vi "Log DB.vi"(8 "error in (no error)":errorcluster, 11 "Class 2 in":refnum<class "Class 2.lvclass">) -> (0 "error out":errorcluster, 3 "Class 2 out":refnum<class "Class 2.lvclass">)   [LabVIEW 2019, in "Class 2.lvclass"]
uses:
  Class 2.lvclass
  Class 2.lvclass/Class 2.ctl
  <vilib>/addons/database/Connection.llb/DB Tools Open Connec (Path).vi
  <vilib>/addons/database/NI_Database_API.lvlib
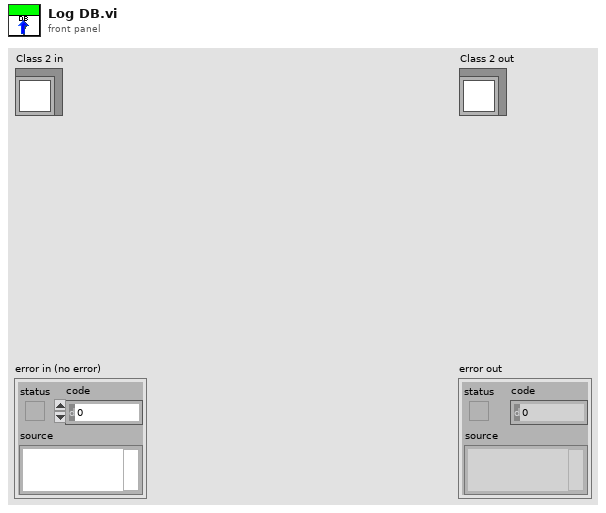
[diagram p1: front panel]
types:
  T1 = cluster{"Modelo":string, "date/time string":string, "Dato1":string, "Dato2":dbl}
  T2 = typedef "NI_Database_API.lvlib/Conn ObjectReference.ctl" = refnum<k1>
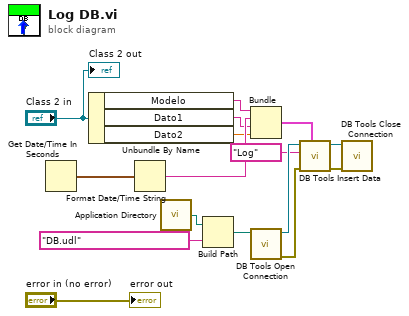
[diagram p0: block diagram]
diagram:
  n1 = Get Date/Time In Seconds() -> (seconds since 1Jan1904=w15:timestamp)
  n2 = Unbundle By Name("Class 2 in") -> ("Modelo"=w3:string, "Dato1"=w2:string, "Dato2"=w1:dbl)
  n3 = Format Date/Time String(seconds (now)=w15) -> (date/time string=w12:string)  [unwired: 2 in]
  n4 = call <vilib>:"Application Directory.vi"() -> ("Application Directory"=w7:path)
  n5 = Build Path(base path=w7, name or relative path="DB.udl") -> (appended path=w5:path)
  n6 = Bundle("Modelo"=w3, "date/time string"=w12, "Dato1"=w2, "Dato2"=w1) -> (w8:T1)  [unwired: 1 in]
  n7 = call-poly <vilib>:"DB Tools Open Connection.vi"("connection information"=w5) -> ("error out"=w11:errorcluster, "connection reference"=w10:T2)  [unwired: 7 in]
  n8 = call <vilib>:"DB Tools Insert Data.vi"("data"=w8, "error in (no error)"=w11, "table"="Log", "connection reference"=w10) -> ("error out"=w14:errorcluster, "connection reference out"=w13:T2)  [unwired: 6 in]
  n9 = call <vilib>:"DB Tools Close Connection.vi"("error in (no error)"=w14, "connection reference"=w13) -> ()  [unwired: 5 in, 1 out]
  "error out" <- "error in (no error)"
  "Class 2 out" <- "Class 2 in"
